vi "update menu frequency.vi"(9 "data rate":variant, 11 "userInterface":T1) -> ()   [LabVIEW 2018]
uses:
  type defs/UI loop data.ctl
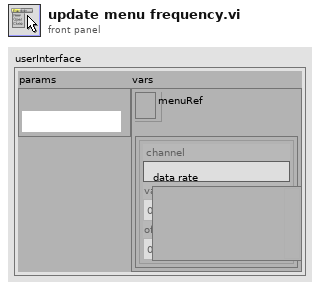
[diagram p1: front panel]
types:
  T1 = typedef "UI loop data.ctl" = cluster{"params":cluster{"channelConfigPath":path}, "vars":cluster{"menuRef":refnum<k9>, "channelOffsets":cluster{"channel":string, "value":dbl, "offset":dbl}[]}}
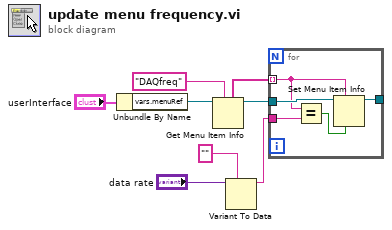
[diagram p0: block diagram]
diagram:
  n1 = Unbundle By Name("userInterface") -> ("vars.menuRef"=w7:refnum<k9>)
  n2 = Get Menu Item Info(7:"DAQfreq" ("item tag"), 11:w7) -> (3:w4:refnum<k9>, 5:w5:string[])  [unwired: 1 in, 5 out]
  n3 = Variant To Data(type="" ("item tag"), Variant="data rate") -> (data=w1:string)  [unwired: 1 in, 1 out]
  n4 = for {
    tunnel: w5 -> [w11] mode=indexing
    tunnel: w4 -> [w13]
    tunnel: [w12] -> _
    tunnel: w1 -> [w10]
    n5 = Equal?(x=w11, y=w10) -> (x = y?=w9:bool)
    n6 = Set Menu Item Info(6:w9, 7:w11, 11:w13) -> (3:w12:refnum<k9>)  [unwired: 4 in, 1 out]
  }
